vi "VIE.Module.Queued Message Handler.dqClass_NotAReferenceConstant.vi"() -> (0 "reference":T1)   [LabVIEW 2010, in "VIE.Module.Queued Message Handler.QueuedMessageHandler.dqGOOPClass.lvlib"]
doc: "Returns a refnum whose value is Not A Refnum. You can use this refnum as an output from structures and subVIs when an error occurs."
uses:
  VIE.Module.Queued Message Handler.QueuedMessageHandler.dqGOOPClass.lvlib
  VIE.Module.Queued Message Handler.dqClass_ObjectReference.ctl
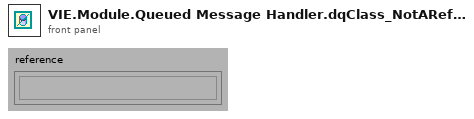
[diagram p1: front panel]
types:
  T1 = typedef "VIE.Module.Queued Message Handler.QueuedMessageHandler.dqGOOPClass.lvlib/VIE.Module.Queued Message Handler.dqClass_ObjectReference.ctl" = refnum<k1>
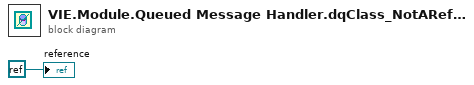
[diagram p0: block diagram]
diagram:
  "reference" <- refnum<k0> refnum
